vi "SerialReadLine.vi"(8 "error in":errorcluster, 11 "VISA resource name in":refnum<visa-resource-name>) -> (0 "error out":errorcluster, 2 "String":string, 3 "VISA resource name out":refnum<visa-resource-name>)   [LabVIEW 2017]
panel:
  out "Elapsed Time (s)":dbl
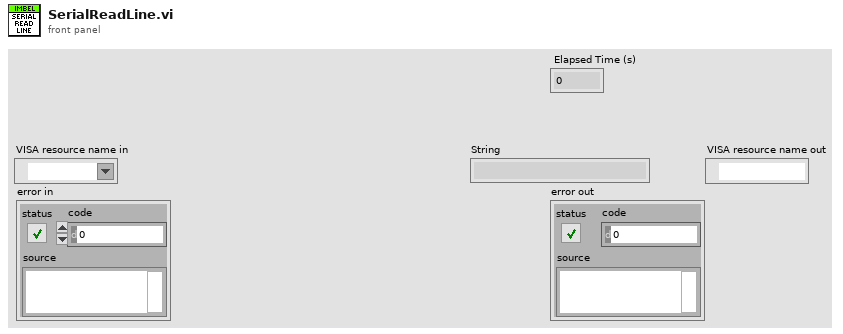
[diagram p1: front panel]
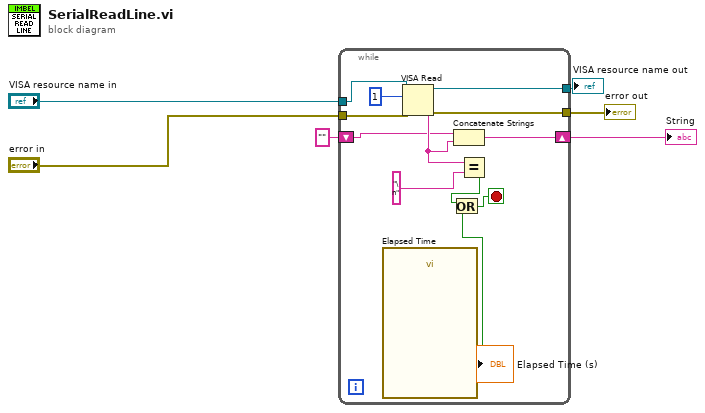
[diagram p0: block diagram]
diagram:
  n1 = while {
    tunnel: "error in" -> [w18]
    tunnel: [w16] -> w4
    tunnel: [w15] -> w5
    shift-right: [w14] -> w6
    shift-left: "" -> [w12]
    tunnel: "VISA resource name in" -> [w11]
    stop <- w8 stop-if-true
    n2 = call "Elapsed Time"() -> ("Elapsed Time (s)"=→"Elapsed Time (s)":dbl, "Time has Elapsed"=w9:bool)  [unwired: 12 in, 6 out]
    n3 = VISA Read(VISA resource name=w11, byte count=u32 1, error in (no error)=w18) -> (VISA resource name out=w16:refnum<visa-resource-name>, read buffer=w13:string, error out=w15:errorcluster)  [unwired: 1 out]
    n4 = Concatenate Strings(w12, w13) -> (w14:string)
    n5 = Equal?(x=w13, y="\n" ("String 2")) -> (x = y?=w10:bool)
    n6 = Or(x=w10, y=w9) -> (x .or. y?=w8:bool)
  }
  "String" <- w6
  "error out" <- w5
  "VISA resource name out" <- w4
